vi "RunAdjustFP.vi"(8 "error in":errorcluster) -> (0 "error out":errorcluster)   [LabVIEW 2023]
uses:
  <vilib>/Wiresmith Technology/G CLI/CLI Class/CLI.lvclass
  _Adjust FP VIs/Adjust FP VIs.lvlib
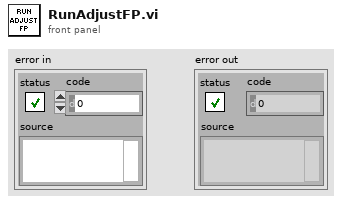
[diagram p1: front panel]
types:
  T1 = enum32{"Invalid", "Standard", "Closed", "Hidden", "Minimized", "Maximized"}
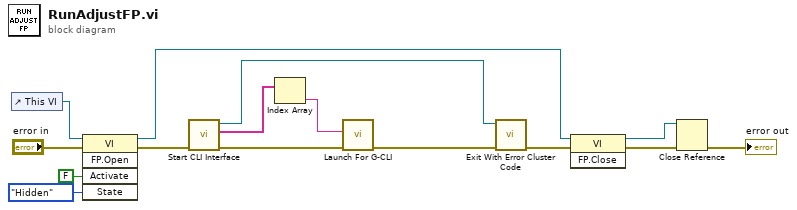
[diagram p0: block diagram]
diagram:
  n1 = control-ref of="This VI"() -> (w10:refnum<vi>)
  n2 = invoke class="VI" method="FP.Open"(reference=w10, error in="error in", "Activate"=FALSE ("Activate?"), "State"=T1."Hidden") -> (reference out=w5:refnum<vi>, error out=w11:errorcluster)  [unwired: 1 in, 3 out]
  n3 = call <vilib>:"Start CLI Interface.vi"("error in (no error)"=w11) -> ("error out"=w14:errorcluster, "Custom Parameters"=w15:string[], "CLI out"=w3:refnum<class "CLI.lvclass">)  [unwired: 7 in, 1 out]
  n4 = Index Array(array=w15) -> (element=w13:string)  [unwired: 1 in]
  n5 = call "Launch For G-CLI.vi"("error in"=w14, "Argument"=w13) -> ("error out"=w2:errorcluster)  [unwired: 9 in]
  n6 = call <vilib>:"Exit With Error Cluster Code.vi"("error in (no error)"=w2, "CLI in"=w3) -> ("error out"=w1:errorcluster)  [unwired: 9 in]
  n7 = invoke class="VI" method="FP.Close"(reference=w5, error in=w1) -> (reference out=w4:refnum<vi>, error out=w7:errorcluster)  [unwired: 1 in, 1 out]
  n8 = Close Reference(reference=w4, error in (no error)=w7) -> (error out=→"error out":errorcluster)
